vi "FTW-JSON-Integer-AtomicIncrement.vi"(0 "JSON":T2, 5 "Path to Integer":string, 7 "Increment":i64=1, 11 "error in":errorcluster) -> (4 "JSON out":T2, 6 "Original Element Type":T1, 8 "New Value":i64, 15 "error out":errorcluster)   [LabVIEW 2015]
uses:
  core/type/FTW-Type-JSON.ctl
  FTW-JSON-Type.ctl
  core/FTW-JSON-Core-Type.ctl
panel:
  # "Inputs"
  # "Outputs"
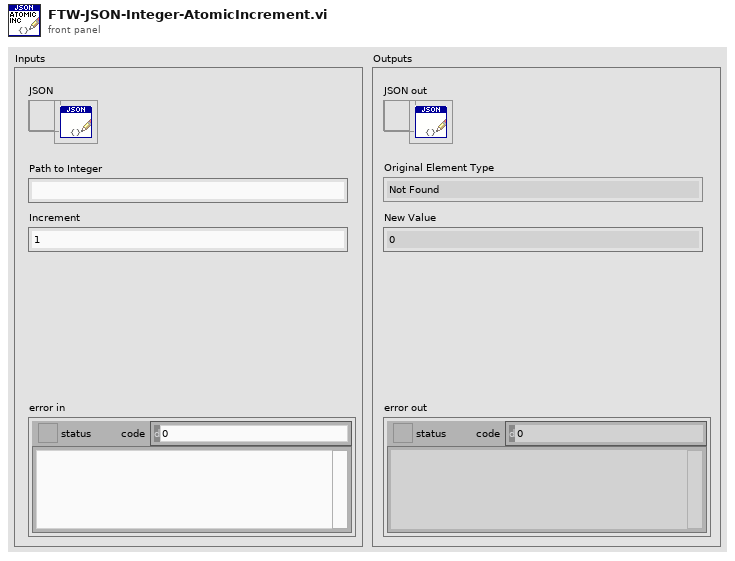
[diagram p1: front panel]
types:
  T1 = typedef "FTW-JSON-Type.ctl" = enum8{"Not Found", "Object", "Array", "String", "Number", "Boolean", "null"}
  T2 = typedef "FTW-Type-JSON.ctl" = refnum<data-value>
  T3 = typedef "FTW-JSON-Core-Type.ctl" = enum8{"Object", "Array", "String", "Integer", "Floating Point", "true", "false", "null", "undefined"}
  T4 = enum8{"<invalid>", "iB", "iW", "iL", "iQ", "uB", "uW", "uL", "uQ", "fS", "fD", "fX", "cS", "cD", "cX"}
  T5 = cluster{"FTW-CodeGen-Type":enum16{"FTW-JSON"}, "Object":i64, "EncodingFlags":i64, "DecodingFlags":i64}
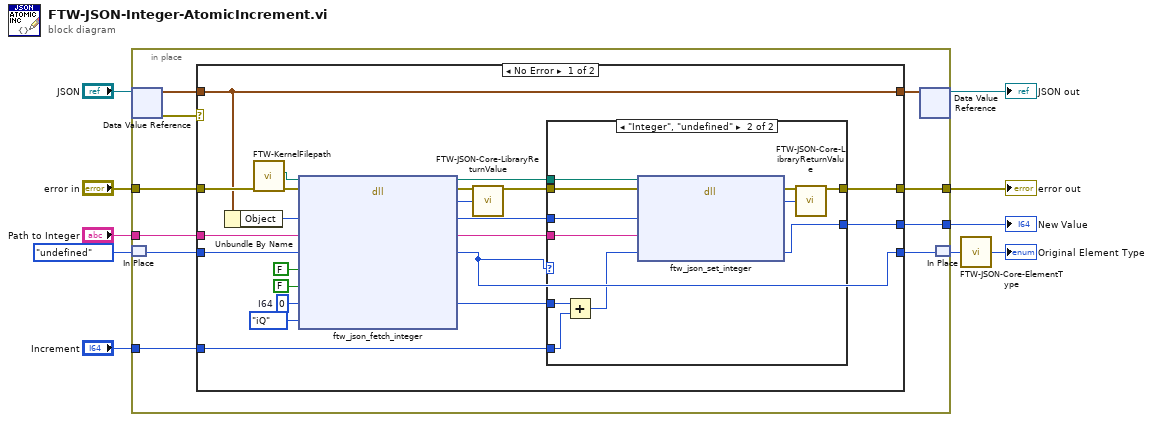
[diagram p0: block diagram]
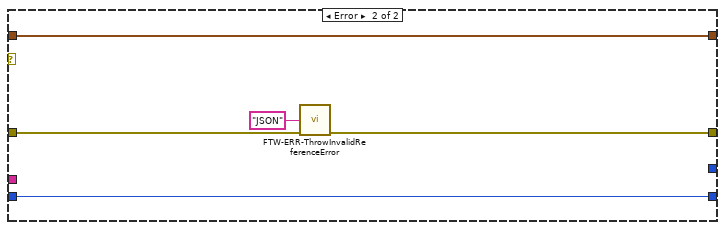
[diagram p3: hidden frame]
diagram:
  n1 = in-place {
    in-place-border: "error in" -> [w16]
    in-place-border: [w17] -> w10
    in-place-border: "Path to Integer" -> [w20]
    in-place-border: "Increment" -> [w18]
    in-place-border: [w11] -> w3
    n2 = in-place-dvr #1("JSON") -> (w19:T5, w14:errorcluster)
    n3 = in-place-match #2(FTW-JSON-Core-Type."undefined" ("JSON Type")) -> (w13:T3)
    n4 = case shown="No Error" w14 {
      tunnel: w20 -> [w29 _]
      tunnel: w19 -> [w41 w59]
      tunnel: w18 -> [w21 _]
      tunnel: [w27 w56] -> w17
      tunnel: w16 -> [w42 w57]
      tunnel: [w41 w59] -> w15
      tunnel: w13 -> [w38 w55]
      tunnel: [w23 w55] -> w12
      tunnel: [w24 _] -> w11
      frame No Error {
        w37 = i64 0  # I64
        n5 = Unbundle By Name(w41) -> ("Object"=w28:i64)
        n6 = call "FTW-KernelFilepath.vi"("error in"=w42) -> ("error out"=w34:errorcluster, "Library Filepath"=w35:path)  [unwired: 8 in, 1 out]
        n7 = dll-call lib="?" fn="ftw_json_fetch_integer"(path in=w35, error in=w34, "JSON Element"=w28, "JSON Path"=w29, "Actual JSON Type"=w38, "Consume?"=FALSE, "Is Flattened?"=FALSE, "Integer Value"=w37, "Integer Type Code"=T4."iQ" ("Scalar NumType")) -> (path out=w30:path, error out=w31:errorcluster, "Return Code"=w32:i64, "JSON Element"=w26:i64, "JSON Path"=w25:string, "Actual JSON Type"=w23:T3, "Integer Value"=w22:i64)  [unwired: 4 in]
        n8 = call "FTW-JSON-Core-LibraryReturnValue.vi"("error in"=w31, "Return Code"=w32) -> ("error out"=w40:errorcluster)  [unwired: 13 in]
        n9 = case shown="\"Integer\", \"undefined\"" w23 {
          tunnel: w40 -> [w43 w54]
          tunnel: w30 -> [_ w53]
          tunnel: [w43 w51] -> w27
          tunnel: w26 -> [_ w49]
          tunnel: w25 -> [_ w48]
          tunnel: [_ w47] -> w24
          tunnel: w22 -> [_ w46]
          tunnel: w21 -> [_ w45]
          frame Default {
          }
          frame "Integer", "undefined" {
            n10 = Add(x=w46, y=w45) -> (x+y=w44:i64)
            n11 = dll-call lib="?" fn="ftw_json_set_integer"(path in=w53, error in=w54, "JSON Object Pointer"=w49, "Key"=w48, "New Value"=w44) -> (error out=w52:errorcluster, "Return Value"=w50:i64, "New Value"=w47:i64)  [unwired: 3 in, 1 out]
            n12 = call "FTW-JSON-Core-LibraryReturnValue.vi"("error in"=w52, "Return Code"=w50) -> ("error out"=w51:errorcluster)  [unwired: 13 in]
          }
        }
      }
      frame Error {
        n13 = call "FTW-ERR-ThrowInvalidReferenceError.vi"("Reference Type"="JSON", "error in"=w57) -> ("error out"=w56:errorcluster)  [unwired: 13 in]
      }
    }
    n14 = in-place-dvr #1(w15) -> (→"JSON out":T2)  [unwired: 1 out]
    n15 = in-place-match #2(w12) -> (w2:T3)
  }
  "error out" <- w10
  "New Value" <- w3
  n16 = call "FTW-JSON-Core-ElementType.vi"("Core Type"=w2) -> ("JSON Element Type"=→"Original Element Type":T1)
